vi "exchangeData_VNA.vi"() -> ()   [LabVIEW 2022 SP3]
doc: "Dieses VI demonstriert, wie eine einfache TCP-Verbindung hergestellt wird und Daten an einen festgelegten Port gesendet werden. Nach dem Senden der Daten wird die Verbindung beendet. Das VI hält an, wenn die TCP-Verbindung unterbrochen wird.\n\nBei den gesendeten Daten handelt es sich um ein Array aus drei Signalverläufen.\n\n<B>Hinweis:</B> Es wird das VI \"Simple Data Client.vi\" benötigt, das sich in derselben Bibliothek befindet."
uses:
  <vilib>/Utility/error.llb/DialogType.ctl
  <instrlib>/Anritsu MS464X Series/Anritsu MS464X Series.lvlib
panel:
  out "save directory":string
  in  "VISA resource name":refnum<visa-resource-name>
  out "Data from Matlab":string
  out "Data to Matlab":string
  in  "Stopp Communication":bool
  in  "Port":u16=2057 caption="Port to Connect" min=1025 step=1
  in  "IP-Addresse":string="localhost" caption="IP-Adresse"
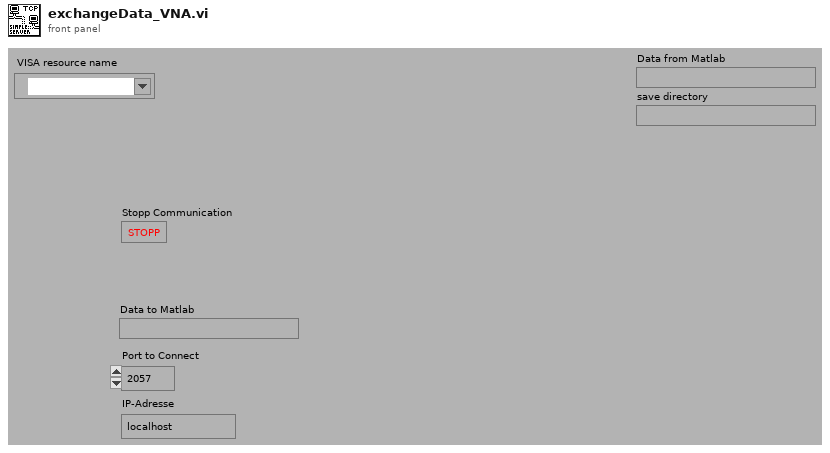
[diagram p1: front panel]
types:
  T1 = enum16{"open", "replace", "create", "open or create", "replace or create", "replace or create with confirmation"}
  T2 = enum16{"Standard", "Buffered", "CRLF", "Immediate"}
  T3 = typedef "DialogType.ctl" = u16
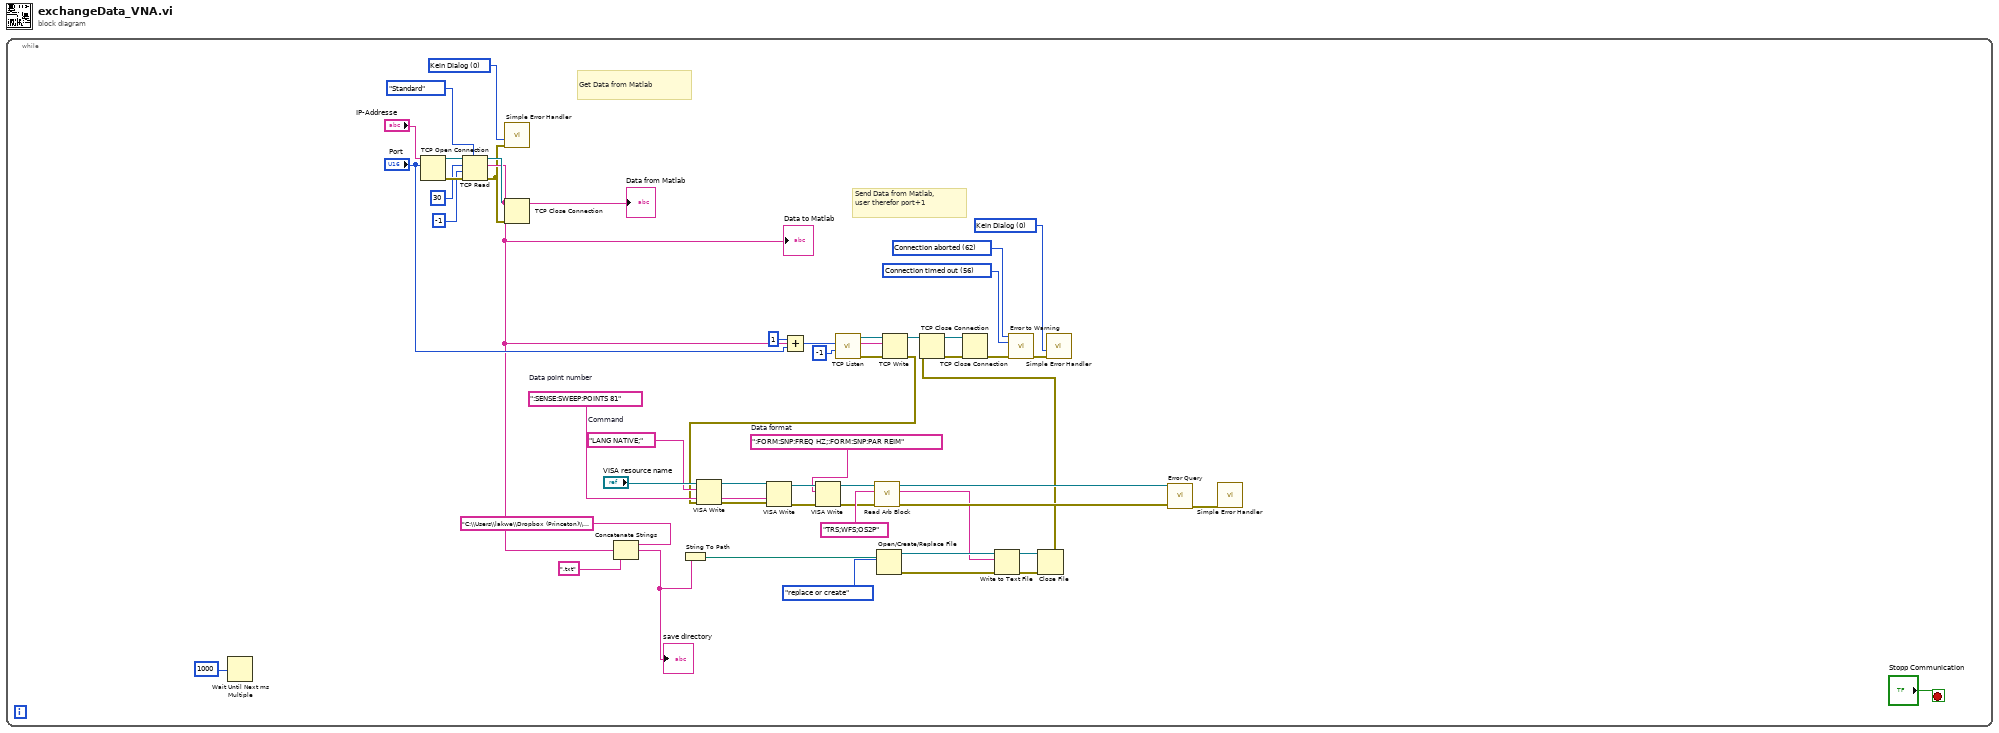
[diagram p0: block diagram]
diagram:
  n1 = while {
    stop <- "Stopp Communication" stop-if-true
    w13 = ":FORM:SNP:FREQ HZ;:FORM:SNP:PAR REIM"  # Data format
    w16 = ":SENSE:SWEEP:POINTS 81"  # Data point number
    w18 = "LANG NATIVE;"  # Command
    w30 = T3 0 items=["Kein Dialog", "OK-Meldung", "Dialog zum Fortsetzen oder Anhalten", "OK-Meldung + Warnungen", "Weiter/Stopp + Warnung"] ("type of dialog (OK msg:1)")
    w34 = 56 items=["No Error", "Argument Error", "Memory Full", "Out of Zone", "End of File", "File Already Open", "Generic File IO Error", "File Not Found", "File Permission Error", "Disk Full", "Duplicate Path", "Too Many Files Open", "Not Enabled", "Resource File Not Found", "Cannot Add Resource", "Resource Not Found", "Image Not Found", "Image Memory Error", "Pen Does Not Exist", "Config Bad Type", "Config Token Not Found", "Config Parse Error", "Config Memory Error", "Bad External Code Format", "Bad External Code Offset", "External Code Not Present", "Null Window", "Destroy Window Mixup", "Null Menu", "Print Aborted", "Bad Print Record", "Print Driver Error", "Windows Error During Print", "Memory Error During Print", "Print Dialog Error", "Generic Print Error", "Invalid Device Refnum", "Device Not Found", "Device Parameter Error", "Device Unit Error", "Can't Open Device", "Device Call Aborted", "Generic Error", "Cancelled By User", "Object ID Too Low", "Object ID Too High", "Object Not In Heap", "Unknown Heap", "Bad DefProc ID", "DefProc Not In Table", "Message Out Of Range", "Null Method", "Unknown Message", "Manager Call Not Supported", "Bad address", "Connection In progress", "Connection timed out", "Connection is already in progress", "Network attribute not supported", "Network error", "Address in use", "System out of memory", "Connection aborted", "Connection refused", "Connection is not connected", "Connection is already connected", "Connection closed", "Initialize error (interapplication manager)", "Bad occurrence", "Wait on unbound occurrence handler", "Occurrence queue overflow", "Bad path", "Semaphore not signaled", "Unrecognized type (interapplication manager)"] ("2nd Error to Convert")
    w35 = 62 items=["No Error", "Argument Error", "Memory Full", "Out of Zone", "End of File", "File Already Open", "Generic File IO Error", "File Not Found", "File Permission Error", "Disk Full", "Duplicate Path", "Too Many Files Open", "Not Enabled", "Resource File Not Found", "Cannot Add Resource", "Resource Not Found", "Image Not Found", "Image Memory Error", "Pen Does Not Exist", "Config Bad Type", "Config Token Not Found", "Config Parse Error", "Config Memory Error", "Bad External Code Format", "Bad External Code Offset", "External Code Not Present", "Null Window", "Destroy Window Mixup", "Null Menu", "Print Aborted", "Bad Print Record", "Print Driver Error", "Windows Error During Print", "Memory Error During Print", "Print Dialog Error", "Generic Print Error", "Invalid Device Refnum", "Device Not Found", "Device Parameter Error", "Device Unit Error", "Can't Open Device", "Device Call Aborted", "Generic Error", "Cancelled By User", "Object ID Too Low", "Object ID Too High", "Object Not In Heap", "Unknown Heap", "Bad DefProc ID", "DefProc Not In Table", "Message Out Of Range", "Null Method", "Unknown Message", "Manager Call Not Supported", "Bad address", "Connection In progress", "Connection timed out", "Connection is already in progress", "Network attribute not supported", "Network error", "Address in use", "System out of memory", "Connection aborted", "Connection refused", "Connection is not connected", "Connection is already connected", "Connection closed", "Initialize error (interapplication manager)", "Bad occurrence", "Wait on unbound occurrence handler", "Occurrence queue overflow", "Bad path", "Semaphore not signaled", "Unrecognized type (interapplication manager)"] ("1st Error to Convert")
    w46 = T3 0 items=["Kein Dialog", "OK-Meldung", "Dialog zum Fortsetzen oder Anhalten", "OK-Meldung + Warnungen", "Weiter/Stopp + Warnung"] ("type of dialog (OK msg:1)")
    # "Send Data from Matlab, user therefor port+1"
    # "Get Data from Matlab"
    n2 = Wait Until Next ms Multiple(millisecond multiple=u32 1000 ("Vielfache von ms")) -> ()  [unwired: 1 out]
    n3 = TCP Open Connection(address="IP-Addresse", remote port or service name="Port") -> (connection ID=w51:refnum<k5>, error out=w50:errorcluster)  [unwired: 3 in]
    n4 = TCP Read(connection ID=w51, bytes to read=30 ("Zu lesende Bytes"), error in (no error)=w50, 7:T2."Standard" ("Modus (Standard)"), 9:-1 ("Timeout in ms (25000)")) -> (connection ID out=w49:refnum<k5>, data out=w4:string, error out=w3:errorcluster)
    "Data to Matlab" <- w4
    "Data from Matlab" <- w4
    n5 = call <vilib>:"Simple Error Handler.vi"("type of dialog (OK msg:1)"=w46, "error in (no error)"=w3) -> ()  [unwired: 3 in, 5 out]
    n6 = TCP Close Connection(connection ID=w49, error in (no error)=w3) -> ()  [unwired: 1 in, 2 out]
    n7 = Concatenate Strings("C:\\Users\\lakwe\\Dropbox (Princeton)\\mmWall2\\code\\VNAData\\081023\\prototype2_0.2V_test6\\txt\\" ("String"), w4, ".txt") -> (w7:string)
    "save directory" <- w7
    n8 = String To Path(string=w7) -> (path=w10:path)
    n9 = Add(x=u16 1, y="Port") -> (x+y=w41:u16)
    n10 = call <vilib>:"TCP Listen.vi"("timeout ms (wait forever: -1)"=-1, "port"=w41) -> ("error out"=w39:errorcluster, "connection ID"=w40:refnum<k5>)  [unwired: 5 in, 3 out]
    n11 = Open/Create/Replace File(file path (use dialog)=w10, operation (0:open)=T1."replace or create") -> (refnum out=w20:refnum<file>, error out=w22:errorcluster)  [unwired: 4 in, 1 out]
    n12 = TCP Write(connection ID=w40, data in=w4, error in (no error)=w39) -> (connection ID out=w31:refnum<k5>, error out=w2:errorcluster)  [unwired: 1 in, 1 out]
    n13 = VISA Write(VISA resource name="VISA resource name", write buffer=w18, error in (no error)=w2) -> (VISA resource name out=w27:refnum<visa-resource-name>, error out=w25:errorcluster)  [unwired: 1 out]
    n14 = VISA Write(VISA resource name=w27, write buffer=w16, error in (no error)=w25) -> (VISA resource name out=w26:refnum<visa-resource-name>, error out=w24:errorcluster)  [unwired: 1 out]
    n15 = VISA Write(VISA resource name=w26, write buffer=w13, error in (no error)=w24) -> (VISA resource name out=w23:refnum<visa-resource-name>, error out=w11:errorcluster)  [unwired: 1 out]
    n16 = call <instrlib>:"Read Arb Block.vi"("error in (no error)"=w11, "Command (\"\")"="TRS;WFS;OS2P", "VISA resource name"=w23) -> ("error out"=w14:errorcluster, "Read Buffer"=w5:string, "VISA resource name out"=w15:refnum<visa-resource-name>)  [unwired: 6 in]
    n17 = Write to Text File(file (use dialog)=w20, text=w5, error in=w22) -> (refnum out=w19:refnum<file>, error out=w21:errorcluster)  [unwired: 1 in, 1 out]
    n18 = Close File(refnum=w19, error in=w21) -> (error out=w1:errorcluster)  [unwired: 1 out]
    n19 = TCP Close Connection(connection ID=w31, error in (no error)=w1) -> (connection ID out=w33:refnum<k5>, error out=w32:errorcluster)  [unwired: 1 in]
    n20 = TCP Close Connection(connection ID=w33, error in (no error)=w32) -> (error out=w37:errorcluster)  [unwired: 1 in, 1 out]
    n21 = call <vilib>:"Error to Warning.vi"("1st Error to Convert"=w35, "2nd Error to Convert"=w34, "error in"=w37) -> ("warning out"=w36:errorcluster)  [unwired: 12 in]
    n22 = call <vilib>:"Simple Error Handler.vi"("type of dialog (OK msg:1)"=w30, "error in (no error)"=w36) -> ()  [unwired: 3 in, 5 out]
    n23 = call <instrlib>:"Error Query.vi"("error in (no error)"=w14, "VISA resource name"=w15) -> ("error out"=w17:errorcluster)  [unwired: 6 in, 3 out]
    n24 = call <vilib>:"Simple Error Handler.vi"("error in (no error)"=w17) -> ()  [unwired: 4 in, 5 out]
  }
